vi "LEP_RV_LaunchProfile.vi"(8 "error in (no error)":errorcluster, 11 "VISA resource name":refnum<visa-resource-name>) -> (0 "error out":errorcluster)   [LabVIEW 2011]
uses:
  LEP_RV_LaunchGlobals.vi
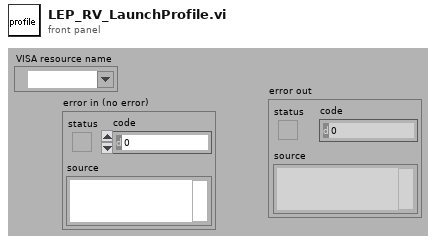
[diagram p1: front panel]
types:
  T1 = enum32{"Bad", "Idle", "Run top level", "Running"}
  T2 = enum32{"Invalid", "Standard", "Closed", "Hidden", "Minimized", "Maximized"}
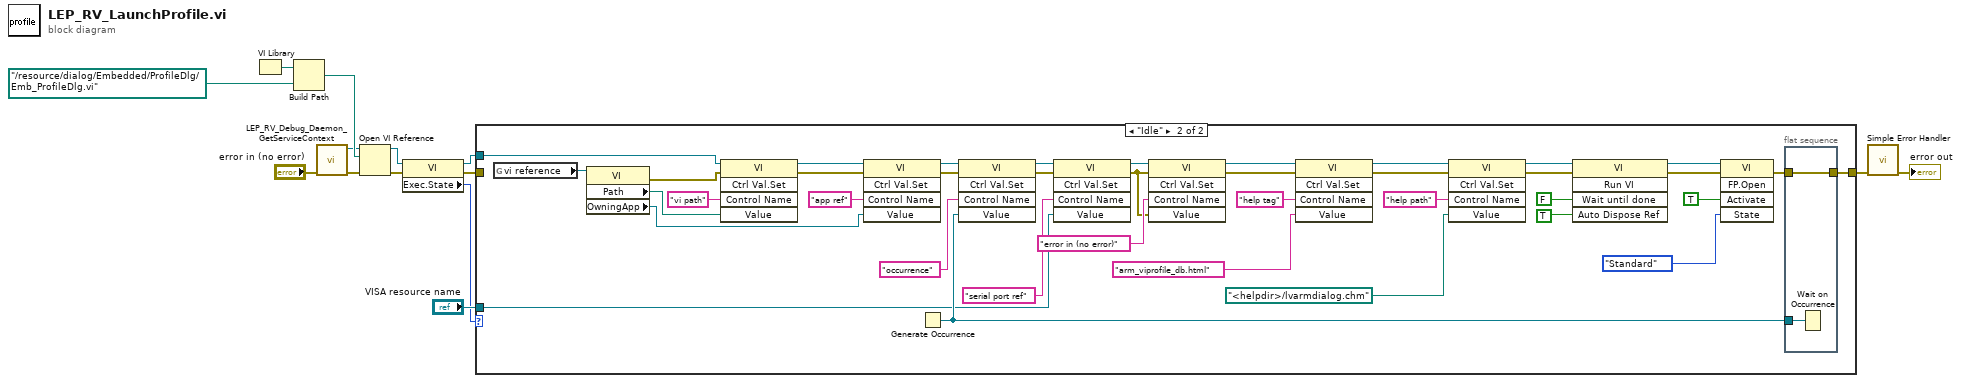
[diagram p0: block diagram]
diagram:
  n1 = VI Library() -> (path=w2:path)
  n2 = Build Path(base path=w2, name or relative path=path "../resource/dialog/Embedded/ProfileDlg/Emb_ProfileDlg.vi") -> (appended path=w11:path)
  n3 = call "LEP_RV_Debug_Daemon_GetServiceContext.vi"("error in"="error in (no error)") -> ("error out"=w9:errorcluster, "service context"=w10:refnum<vi>)  [unwired: 9 out]
  n4 = Open VI Reference(application reference (local)=w10, vi path=w11, error in (no error)=w9) -> (vi reference=w7:refnum<vi>, error out=w8:errorcluster)  [unwired: 3 out]
  n5 = property class="VI"(reference=w7, error in=w8) -> (reference out=w5:refnum<vi>, error out=w6:errorcluster, "Exec.State"=w4:T1)
  n6 = case shown="\"Idle\"" w4 {
    tunnel: [w15 w42] -> w14
    tunnel: "VISA resource name" -> [_ w22]
    tunnel: w5 -> [_ w16]
    tunnel: w6 -> [w15 _]
    frame Default {
    }
    frame "Idle" {
      n7 = global read "LEP_RV_LaunchGlobals.vi" "vi reference"() -> (w20:refnum<vi>)
      n8 = property class="VI"(reference=w20) -> (error out=w17:errorcluster, "Path"=w19:path, "OwningApp"=w18:refnum<vi>)  [unwired: 1 in, 1 out]
      n9 = invoke class="VI" method="Ctrl Val.Set"(reference=w16, error in=w17, "Control Name"="vi path", "Value"=w19) -> (reference out=w49:refnum<vi>, error out=w21:errorcluster)  [unwired: 1 in, 3 out]
      n10 = invoke class="VI" method="Ctrl Val.Set"(reference=w49, error in=w21, "Control Name"="app ref", "Value"=w18) -> (reference out=w48:refnum<vi>, error out=w45:errorcluster)  [unwired: 1 in, 3 out]
      n11 = Generate Occurrence() -> (w46:refnum<k4>)
      n12 = invoke class="VI" method="Ctrl Val.Set"(reference=w48, error in=w45, "Control Name"="occurrence", "Value"=w46) -> (reference out=w47:refnum<vi>, error out=w41:errorcluster)  [unwired: 1 in, 3 out]
      n13 = invoke class="VI" method="Ctrl Val.Set"(reference=w47, error in=w41, "Control Name"="serial port ref", "Value"=w22) -> (reference out=w44:refnum<vi>, error out=w38:errorcluster)  [unwired: 1 in, 3 out]
      n14 = invoke class="VI" method="Ctrl Val.Set"(reference=w44, error in=w38, "Control Name"="error in (no error)", "Value"=w38) -> (reference out=w28:refnum<vi>, error out=w25:errorcluster)  [unwired: 1 in, 3 out]
      n15 = invoke class="VI" method="Ctrl Val.Set"(reference=w28, error in=w25, "Control Name"="help tag", "Value"="arm_viprofile_db.html" ("Control Name")) -> (reference out=w31:refnum<vi>, error out=w32:errorcluster)  [unwired: 1 in, 3 out]
      n16 = invoke class="VI" method="Ctrl Val.Set"(reference=w31, error in=w32, "Control Name"="help path", "Value"=path "<helpdir>/lvarmdialog.chm") -> (reference out=w27:refnum<vi>, error out=w26:errorcluster)  [unwired: 1 in, 3 out]
      n17 = invoke class="VI" method="Run VI"(reference=w27, error in=w26, "Wait until done"=FALSE, "Auto Dispose Ref"=TRUE) -> (reference out=w33:refnum<vi>, error out=w35:errorcluster)  [unwired: 1 in, 3 out]
      n18 = invoke class="VI" method="FP.Open"(reference=w33, error in=w35, "Activate"=TRUE, "State"=T2."Standard") -> (error out=w34:errorcluster)  [unwired: 1 in, 4 out]
      n19 = flat-sequence {
        tunnel: w46 -> [w55]
        tunnel: w34 -> [w54]
        tunnel: [w54] -> w42
        frame #0 {
          n20 = Wait on Occurrence(2:w55) -> ()  [unwired: 3 out]
        }
      }
    }
  }
  n21 = call <vilib>:"Simple Error Handler.vi"("error in (no error)"=w14) -> ("error out"=→"error out":errorcluster)  [unwired: 1 in, 7 out]
